vi "Position.vi"() -> (1 "Z":dbl, 2 "Y":dbl, 3 "X":dbl)   [LabVIEW 2017]
uses:
  <userlib>/HapticSTM/Feedbackless - Testdata/Project/feedbackless.lvproj/Proj/Feedbackless Folder/HapticSTM/HapticSTM.lvlib
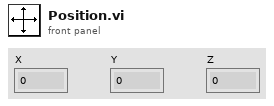
[diagram p1: front panel]
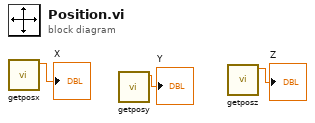
[diagram p0: block diagram]
diagram:
  n1 = call <userlib>:"getposx.vi"() -> ("function return"=→"X":dbl)  [unwired: 11 in]
  n2 = call <userlib>:"getposy.vi"() -> ("function return"=→"Y":dbl)  [unwired: 11 in]
  n3 = call <userlib>:"getposz.vi"() -> ("function return"=→"Z":dbl)  [unwired: 11 in]
